vi "LWXPS_GroupAccelerationSetpointGet.vi"(0 "XPS Reference IN":refnum<k24>, 5 "Group Name":string, 7 "Number of Positioners":i32, 11 "LabVIEW error IN":errorcluster) -> (4 "XPS Reference OUT":refnum<k24>, 6 "Returned error code":i32, 8 "XPS Error String":string, 10 "Setpoint Acceleration":dbl[](array[numeric]), 15 "LabVIEW error OUT":errorcluster)   [LabVIEW 2014]
uses:
  D:/XPSQ8_LabView_Library/Development/Source/Dll/Newport.XPS.CommandInterface.dll
  Dll/Newport.XPS.CommandInterface.dll
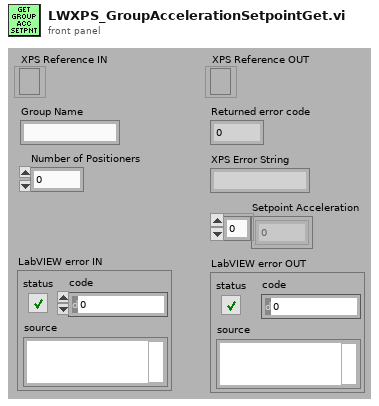
[diagram p1: front panel]
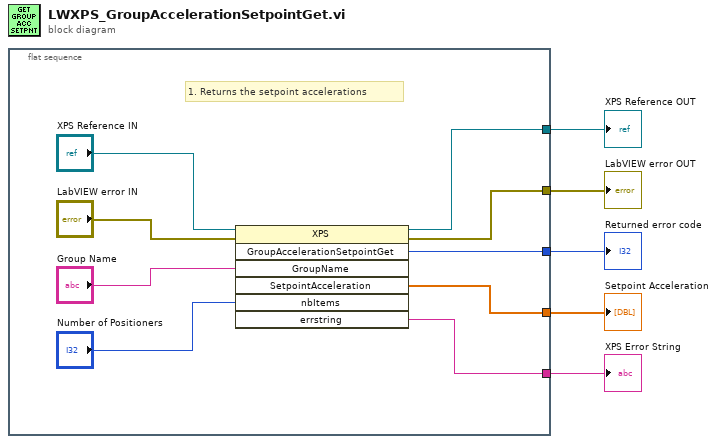
[diagram p0: block diagram]
diagram:
  n1 = flat-sequence {
    tunnel: [w11] -> w5
    tunnel: [w14] -> w4
    tunnel: [w12] -> w3
    tunnel: [w9] -> w2
    tunnel: [w8] -> w1
    frame #0 {
      # "1. Returns the setpoint accelerations"
      n2 = invoke class="XPS" method="GroupAccelerationSetpointGet"(reference="XPS Reference IN", error in="LabVIEW error IN", "GroupName"="Group Name", "nbItems"="Number of Positioners") -> (reference out=w11:refnum<k24>, error out=w14:errorcluster, "GroupAccelerationSetpointGet"=w12:i32, "SetpointAcceleration"=w8:dbl[], "errstring"=w9:string)  [unwired: 3 in, 2 out]
    }
  }
  "XPS Reference OUT" <- w5
  "LabVIEW error OUT" <- w4
  "Returned error code" <- w3
  "XPS Error String" <- w2
  "Setpoint Acceleration" <- w1
